vi "GUI PS Insertion.vi"(6 "PS Graph Selector ALV":T1[](array[typedef]), 9 "PS Graph Selector Vertical":T1[](array[typedef]), 10 "PS Graph Selector Horizontal":T1[](array[typedef])) -> (3 "PS Graph Selector out":T1[](array[typedef]))   [LabVIEW 2011, in "User Interface VIs.lvlib"]
uses:
  User Interface VIs.lvlib
  Types Definitions/Type BPM or PS Selector.ctl
  Type Definitions.lvlib
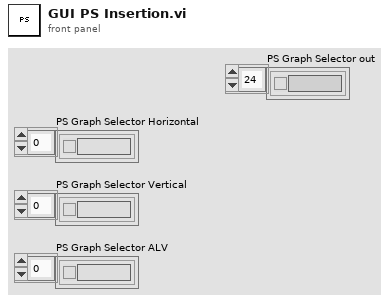
[diagram p1: front panel]
types:
  T1 = typedef "Type Definitions.lvlib/Type BPM or PS Selector.ctl" = cluster{"Name":string, "Active":bool}
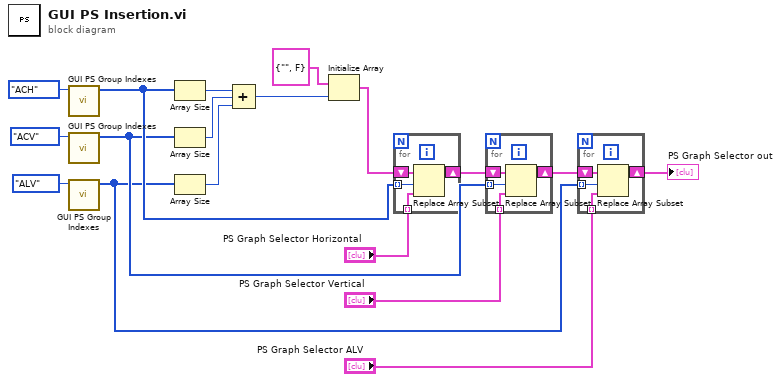
[diagram p0: block diagram]
diagram:
  n1 = call "GUI PS Group Indexes.vi"("PS Group"=enum16{"ACH", "ACV", "ALV"}."ACH") -> ("Indexes"=w12:i32[])  [unwired: 10 in]
  n2 = call "GUI PS Group Indexes.vi"("PS Group"=enum16{"ACH", "ACV", "ALV"}."ACV") -> ("Indexes"=w2:i32[])  [unwired: 10 in]
  n3 = call "GUI PS Group Indexes.vi"("PS Group"=enum16{"ACH", "ACV", "ALV"}."ALV") -> ("Indexes"=w1:i32[])  [unwired: 10 in]
  n4 = Array Size(array=w12) -> (size(s)=w18:i32)
  n5 = Array Size(array=w2) -> (size(s)=w17:i32)
  n6 = Array Size(array=w1) -> (size(s)=w16:i32)
  n7 = Compound Arithmetic op=ADD(w18, w17, w16) -> (w14:i32)
  n8 = Initialize Array(T1 {"Name"="", "Active"=FALSE} ("BPM or PS Selection"), w14) -> (w13:T1[])
  n9 = for {
    tunnel: w12 -> [w21] mode=indexing
    tunnel: "PS Graph Selector Horizontal" -> [w19] mode=indexing
    shift-right: [w20] -> w11
    shift-left: w13 -> [w22]
    n10 = Replace Array Subset(array=w22, new element=w19, index=w21) -> (w20:T1[])
  }
  n11 = for {
    tunnel: w2 -> [w25] mode=indexing
    tunnel: "PS Graph Selector Vertical" -> [w23] mode=indexing
    shift-right: [w24] -> w10
    shift-left: w11 -> [w26]
    n12 = Replace Array Subset(array=w26, new element=w23, index=w25) -> (w24:T1[])
  }
  n13 = for {
    tunnel: w1 -> [w29] mode=indexing
    tunnel: "PS Graph Selector ALV" -> [w28] mode=indexing
    shift-right: [w27] -> w6
    shift-left: w10 -> [w30]
    n14 = Replace Array Subset(array=w30, new element=w28, index=w29) -> (w27:T1[])
  }
  "PS Graph Selector out" <- w6
